vi "Write DefaultCellBGKColor.vi"(8 "error in (no error)":errorcluster, 10 "CellBGKColor":u32(colorbox)=16777215, 11 "DataGridView in":refnum<class "DataGridView.lvclass">) -> (0 "error out":errorcluster, 3 "DataGridView out":refnum<class "DataGridView.lvclass">)   [LabVIEW 2014, in "DataGridView.lvclass"]
uses:
  DataGridView.lvclass
  System.Drawing
  DataGridView.lvclass/DataGridView.ctl
  System.Windows.Forms
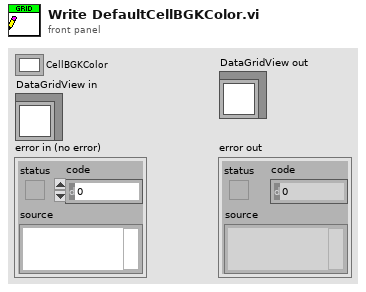
[diagram p1: front panel]
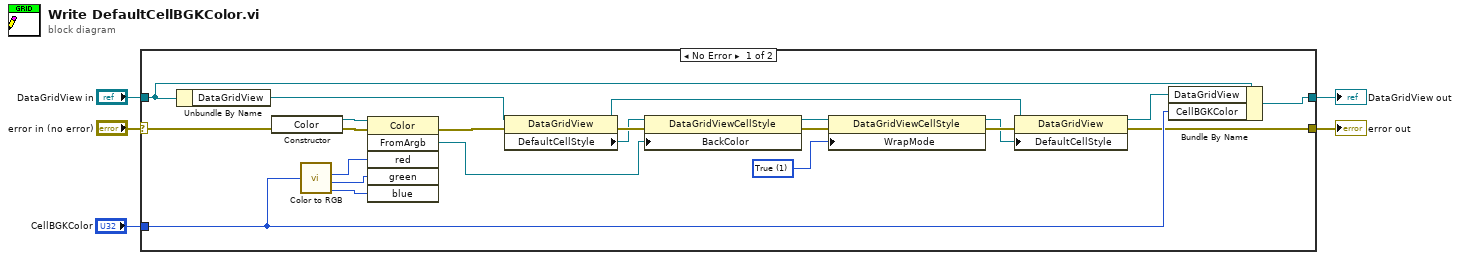
[diagram p0: block diagram]
diagram:
  n1 = case shown="No Error" "error in (no error)" {
    selector: "error in (no error)" -> [w18 w28]
    tunnel: [w11 w28] -> w4
    tunnel: [w27 w29] -> w2
    tunnel: "DataGridView in" -> [w21 w29]
    tunnel: "CellBGKColor" -> [w20 _]
    frame No Error {
      w10 = 1 items=["NotSet", "True", "False"] ("WrapMode")
      n2 = Unbundle By Name(w21) -> ("DataGridView"=w19:refnum<k24>)
      n3 = constructor class="Color"(error in=w18) -> (reference out=w22:refnum<k24>, error out=w23:errorcluster)  [unwired: 2 in, 1 out]
      n4 = call <vilib>:"Color to RGB.vi"("Color"=w20) -> ("R"=w24:u8, "G"=w25:u8, "B"=w26:u8)  [unwired: 1 out]
      n5 = invoke class="Color" method="FromArgb"(reference=w22, error in=w23, "red"=w24, "green"=w25, "blue"=w26) -> (error out=w17:errorcluster, "FromArgb"=w13:refnum<k24>)  [unwired: 1 in, 4 out]
      n6 = property class="DataGridView"(reference=w19, error in=w17) -> (reference out=w16:refnum<k24>, error out=w15:errorcluster, "DefaultCellStyle"=w12:refnum<k24>)
      n7 = property class="DataGridViewCellStyle"(reference=w12, error in=w15, "BackColor"=w13) -> (reference out=w9:refnum<k24>, error out=w8:errorcluster)
      n8 = property class="DataGridViewCellStyle"(reference=w9, error in=w8, "WrapMode"=w10) -> (reference out=w6:refnum<k24>, error out=w7:errorcluster)
      n9 = property class="DataGridView"(reference=w16, error in=w7, "DefaultCellStyle"=w6) -> (reference out=w14:refnum<k24>, error out=w11:errorcluster)
      n10 = Bundle By Name(cluster=w21, "DataGridView"=w14, "CellBGKColor"=w20) -> (w27:refnum<class "DataGridView.lvclass">)
    }
    frame Error {
    }
  }
  "error out" <- w4
  "DataGridView out" <- w2
